vi "ChangeTypeInternalVariables.vi"(8 "error in":errorcluster, 11 "ESC Internal Data Structure":T1={"Test_File"="", "Status"="Done", "RF_Center_Freq"="0", "RF_Gain"="0", "BB_Gain"="0", "Error"="", "file_max"="0", "file_index"="0"}) -> (0 "error out":errorcluster, 3 "ESC Internal Data Structure (with types)":T2={"Test_File"=path "", "Status"="Done", "RF_Center_Freq"=0.0, "RF_Gain"=0.0, "BB_Gain"=0.0, "Error 2"="", "file_max"=0, "file_index"=0})   [LabVIEW 2017]
uses:
  TypeDef/RF Internal Data Structure (types).ctl
  TypeDef/RF Internal Data Structure (string).ctl
  MainVI/GlobalVariableS.vi
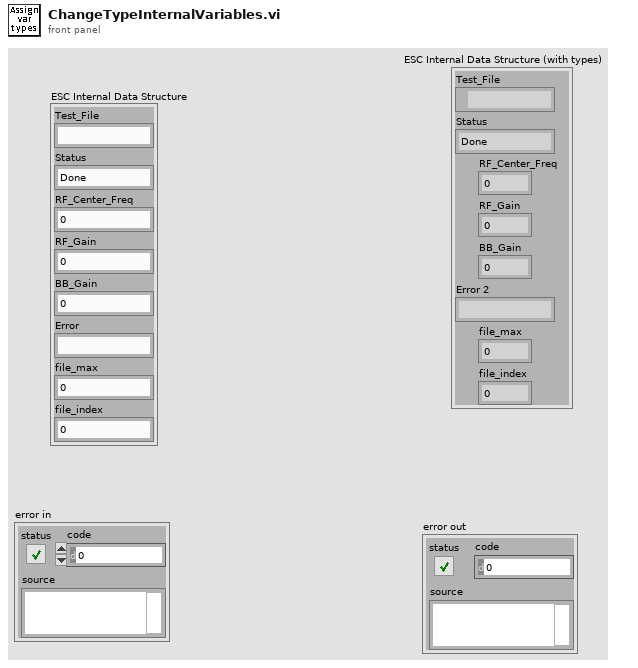
[diagram p1: front panel]
types:
  T1 = typedef "RF Internal Data Structure (string).ctl" = cluster{"Test_File":string, "Status":string, "RF_Center_Freq":string, "RF_Gain":string, "BB_Gain":string, "Error":string, "file_max":string, "file_index":string}
  T2 = typedef "RF Internal Data Structure (types).ctl" = cluster{"Test_File":path, "Status":string, "RF_Center_Freq":dbl, "RF_Gain":dbl, "BB_Gain":dbl, "Error 2":string, "file_max":u64, "file_index":u64}
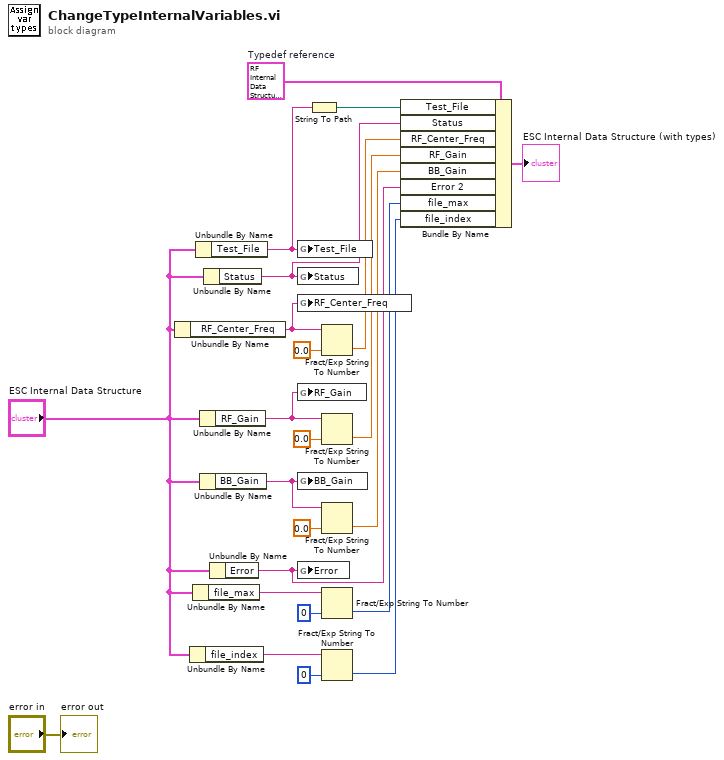
[diagram p0: block diagram]
diagram:
  w23 = T2 {"Test_File"=path "", "Status"="Done", "RF_Center_Freq"=0.0, "RF_Gain"=0.0, "BB_Gain"=0.0, "Error 2"="", "file_max"=0, "file_index"=0}  # Typedef reference
  n1 = Unbundle By Name("ESC Internal Data Structure") -> ("RF_Center_Freq"=w4:string)
  n2 = Unbundle By Name("ESC Internal Data Structure") -> ("file_index"=w10:string)
  n3 = Unbundle By Name("ESC Internal Data Structure") -> ("file_max"=w9:string)
  n4 = Unbundle By Name("ESC Internal Data Structure") -> ("Test_File"=w6:string)
  n5 = Unbundle By Name("ESC Internal Data Structure") -> ("RF_Gain"=w1:string)
  n6 = Unbundle By Name("ESC Internal Data Structure") -> ("BB_Gain"=w3:string)
  n7 = Unbundle By Name("ESC Internal Data Structure") -> ("Status"=w5:string)
  n8 = Unbundle By Name("ESC Internal Data Structure") -> ("Error"=w2:string)
  n9 = global write "GlobalVariableS.vi" "Test_File"(w6) -> ()
  n10 = global write "GlobalVariableS.vi" "Status"(w5) -> ()
  n11 = global write "GlobalVariableS.vi" "RF_Center_Freq"(w4) -> ()
  n12 = global write "GlobalVariableS.vi" "RF_Gain"(w1) -> ()
  n13 = global write "GlobalVariableS.vi" "BB_Gain"(w3) -> ()
  n14 = global write "GlobalVariableS.vi" "Error"(w2) -> ()
  n15 = String To Path(string=w6) -> (path=w19:path)
  n16 = Fract/Exp String To Number(string=w4, default (0 dbl)=0.0 ("default (0 DBL)")) -> (number=w20:dbl)  [unwired: 2 in, 1 out]
  n17 = Fract/Exp String To Number(string=w1, default (0 dbl)=0.0 ("default (0 DBL)")) -> (number=w21:dbl)  [unwired: 2 in, 1 out]
  n18 = Fract/Exp String To Number(string=w3, default (0 dbl)=0.0 ("default (0 DBL)")) -> (number=w18:dbl)  [unwired: 2 in, 1 out]
  n19 = Fract/Exp String To Number(string=w9, default (0 dbl)=u64 0 ("default (0 DBL)")) -> (number=w16:u64)  [unwired: 2 in, 1 out]
  n20 = Fract/Exp String To Number(string=w10, default (0 dbl)=u64 0 ("default (0 DBL)")) -> (number=w14:u64)  [unwired: 2 in, 1 out]
  n21 = Bundle By Name(cluster=w23, "Test_File"=w19, "Status"=w5, "RF_Center_Freq"=w20, "RF_Gain"=w21, "BB_Gain"=w18, "Error 2"=w2, "file_max"=w16, "file_index"=w14) -> (→"ESC Internal Data Structure (with types)":T2)
  "error out" <- "error in"
